vi "DeleteMeSaveTests.vi"() -> ()   [LabVIEW 2019]
uses:
  DAQ_cRIO9073/DAQ/controls/UI Save FGV.ctl
panel:
  out "tdms file out":refnum<k34>
  out "error out":errorcluster
  in  "Name":string="Test"
  in  "State":T1
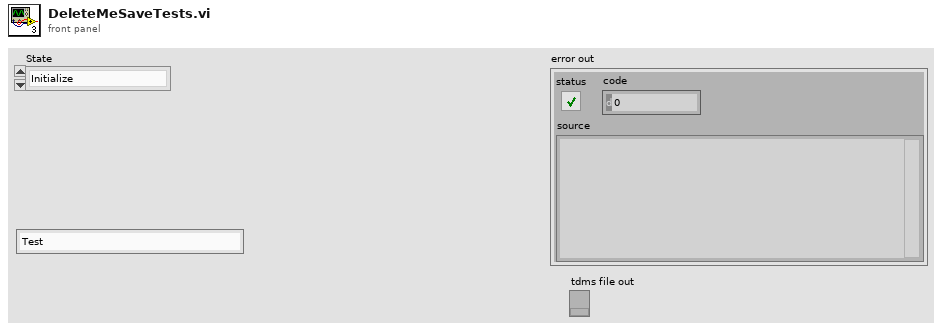
[diagram p1: front panel]
types:
  T1 = typedef "UI Save FGV.ctl" = enum16{"Initialize", "Write", "Pass", "Kill"}
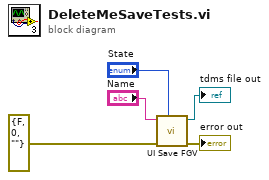
[diagram p0: block diagram]
diagram:
  n1 = call "UI Save FGV.vi"("State"="State", "error in (no error)"=errorcluster {"status"=FALSE, "code"=0, "source"=""}, "Name"="Name") -> ("error out"=→"error out":errorcluster, "tdms file out"=→"tdms file out":refnum<k34>)  [unwired: 6 in, 1 out]
